vi "FindAliasIPAddress.vi"(4 "alias":string, 5 "hosts":T1[](array[typedef]), 6 "error in":errorcluster) -> (0 "error out":errorcluster, 3 "IP address":string)   [LabVIEW 2014, in "Autodetect.lvlib"]
uses:
  Autodetect.lvlib
  TypeDefs/HostTD.ctl
  TypeDefs/UDP_HostinfoTD.ctl
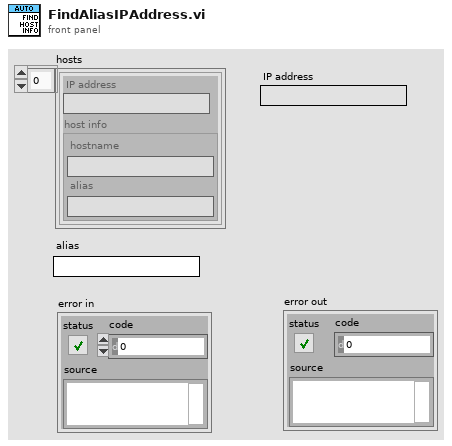
[diagram p1: front panel]
types:
  T1 = typedef "Autodetect.lvlib/HostTD.ctl" = cluster{"IP address":string, "host info":T2}
  T2 = typedef "Autodetect.lvlib/UDP_HostinfoTD.ctl" = cluster{"hostname":string, "alias":string}
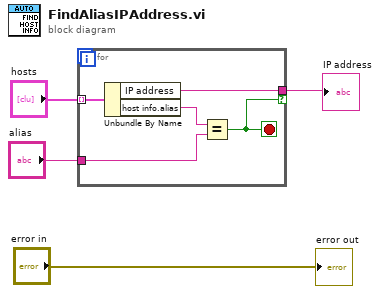
[diagram p0: block diagram]
diagram:
  n1 = for {
    tunnel: "hosts" -> [w9] mode=indexing
    tunnel: "alias" -> [w6]
    tunnel: [w8] -> w2 if=w5
    stop <- w5 stop-if-true
    n2 = Unbundle By Name(w9) -> ("IP address"=w8:string, "host info.alias"=w7:string)
    n3 = Equal?(x=w7, y=w6) -> (x = y?=w5:bool)
  }
  "IP address" <- w2
  "error out" <- "error in"
